vi "save_data.vi"(8 "bboxes":T1(array[cluster]), 9 "classes":string[](array[string]), 10 "Dataset path":path, 11 "Image path":path) -> ()   [LabVIEW 2024]
uses:
  <vilib>/Utility/file.llb/Write Delimited Spreadsheet (string).vi
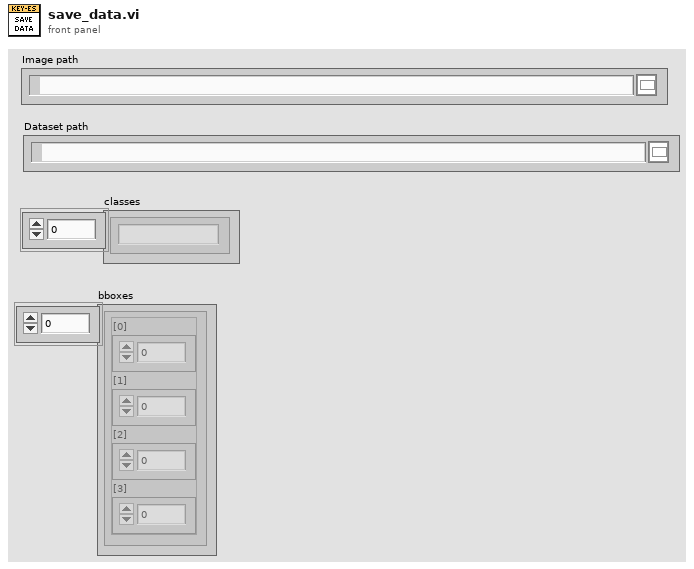
[diagram p1: front panel]
types:
  T1 = cluster{"[0]":dbl, "[1]":dbl, "[2]":dbl, "[3]":dbl}[]
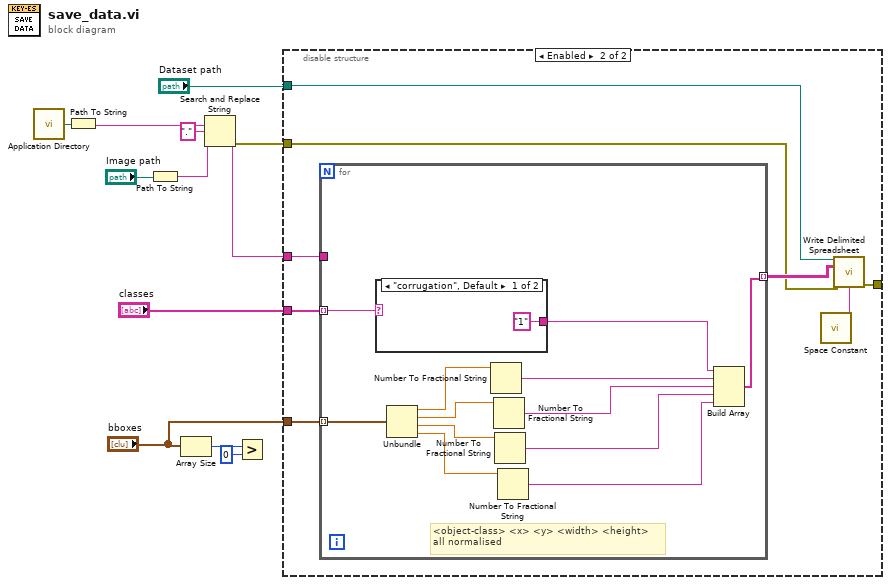
[diagram p0: block diagram]
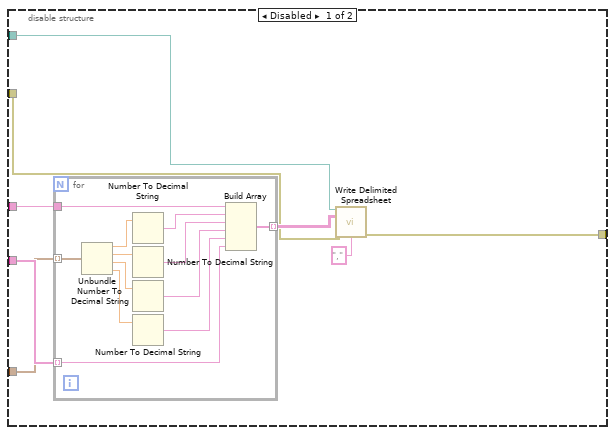
[diagram p2: hidden frame]
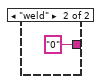
[diagram p3: hidden frame]
diagram:
  n1 = call <vilib>:"Application Directory.vi"() -> ("Application Directory"=w8:path)
  n2 = Path To String(path=w8) -> (string=w6:string)
  n3 = Path To String(path="Image path") -> (string=w7:string)
  n4 = Array Size(array="bboxes") -> (size(s)=w11:i32)
  n5 = Search and Replace String(input string=w7, search string=w6, replace string="." ("replace string (\"\")")) -> (result string=w4:string, error out=w3:errorcluster)  [unwired: 5 in, 2 out]
  n6 = Greater?(x=w11, y=0) -> ()  [unwired: 1 out]
  n7 = disable-structure shown="Enabled" {
    disable-tunnel: "classes" -> [w19 w40]
    disable-tunnel: "bboxes" -> [w18 w39]
    disable-tunnel: w4 -> [w17 w38]
    disable-tunnel: w3 -> [w15 w36]
    disable-tunnel: [w14 w35] -> _
    disable-tunnel: "Dataset path" -> [w13 w33]
    frame Disabled {
      n8 = for {
        tunnel: w19 -> [w26] mode=indexing
        tunnel: w18 -> [w31] mode=indexing
        tunnel: w17 -> [w32]
        tunnel: [w21] -> w16 mode=indexing
        n9 = Unbundle(w31) -> ("[0]"=w29:dbl, "[1]"=w28:dbl, "[2]"=w27:dbl, "[3]"=w30:dbl)
        n10 = Number To Decimal String(number=w29) -> (decimal integer string=w22:string)  [unwired: 1 in]
        n11 = Number To Decimal String(number=w28) -> (decimal integer string=w23:string)  [unwired: 1 in]
        n12 = Number To Decimal String(number=w27) -> (decimal integer string=w24:string)  [unwired: 1 in]
        n13 = Number To Decimal String(number=w30) -> (decimal integer string=w25:string)  [unwired: 1 in]
        n14 = Build Array(w32, w22, w23, w24, w25, w26) -> (w21:string[])
      }
      n15 = call-poly <vilib>:"Write Delimited Spreadsheet.vi"("file path (dialog if empty)"=w13, "2D data"=w16, "error in (no error)"=w15, "delimiter (\\t)"="," ("delimiter (\\t)")) -> ("error out"=w14:errorcluster)  [unwired: 10 in, 1 out]
    }
    frame Enabled {
      n16 = for {
        tunnel: w40 -> [w42] mode=indexing
        tunnel: w39 -> [w52] mode=indexing
        tunnel: w38 -> [_]
        tunnel: [w47] -> w37 mode=indexing
        # "<object-class> <x> <y> <width> <height>\nall normalised"
        n17 = case shown="\"corrugation\", Default" w42 {
          tunnel: ["1" ("element") "0" ("element")] -> w41
          frame "corrugation", Default {
          }
          frame "weld" {
          }
        }
        n18 = Unbundle(w52) -> ("[0]"=w43:dbl, "[1]"=w44:dbl, "[2]"=w45:dbl, "[3]"=w46:dbl)
        n19 = Number To Fractional String(number=w43) -> (F-format string=w48:string)  [unwired: 3 in]
        n20 = Number To Fractional String(number=w44) -> (F-format string=w49:string)  [unwired: 3 in]
        n21 = Number To Fractional String(number=w45) -> (F-format string=w50:string)  [unwired: 3 in]
        n22 = Number To Fractional String(number=w46) -> (F-format string=w51:string)  [unwired: 3 in]
        n23 = Build Array(w41, w48, w49, w50, w51) -> (w47:string[])
      }
      n24 = call <vilib>:"Space Constant.vi"() -> ("String"=w34:string)
      n25 = call-poly <vilib>:"Write Delimited Spreadsheet.vi"("file path (dialog if empty)"=w33, "2D data"=w37, "error in (no error)"=w36, "delimiter (\\t)"=w34) -> ("error out"=w35:errorcluster)  [unwired: 10 in, 1 out]
    }
  }
